vi "Test_WriteValue_InvalidRefnum_Error.vi"(8 "error in (no error)":errorcluster, 11 "TestCase in":refnum<class "TestTerminalCaptionBinding.lvclass">) -> (0 "error out":errorcluster, 3 "TestCase out":refnum<class "TestTerminalCaptionBinding.lvclass">)   [LabVIEW 2017, in "TestTerminalCaptionBinding.lvclass"]
uses:
  TestTerminalCaptionBinding.lvclass
  Source/Concrete/TerminalCaptionBinding/TerminalCaptionBinding.lvclass
  C:/Git/composed-transport/Source/ITransport/ITransport.lvclass
  Source/ITransport/ITransport.lvclass
panel:
  out "Return Error":errorcluster
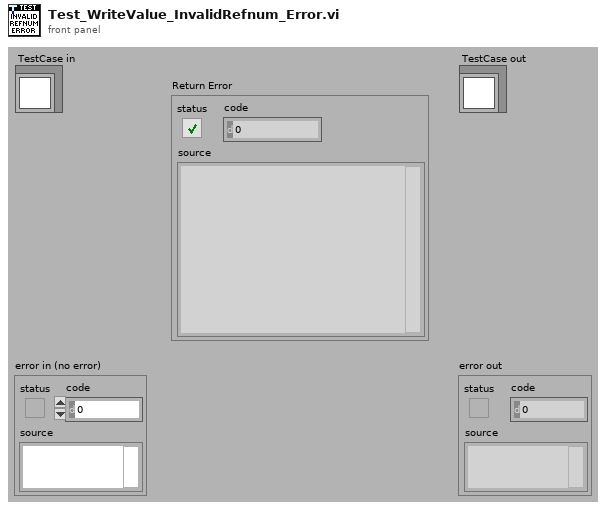
[diagram p1: front panel]
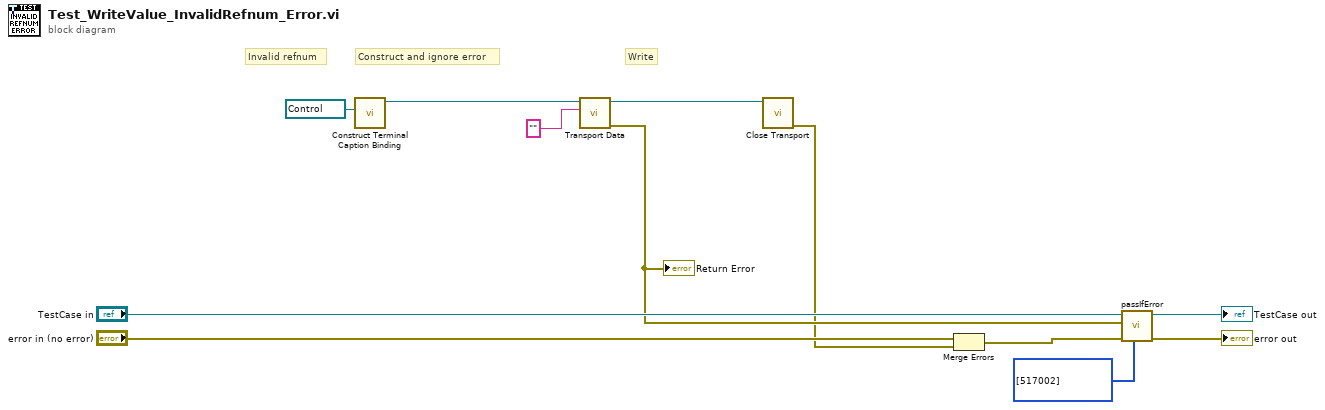
[diagram p0: block diagram]
diagram:
  # "Invalid refnum"
  # "Write"
  # "Construct and ignore error"
  n1 = call "Construct Terminal Caption Binding.vi"("Ctl Refnum"=refnum<vi> refnum) -> ("TerminalCaptionBinding"=w9:refnum<class "TerminalCaptionBinding.lvclass">)  [unwired: 9 in, 1 out]
  n2 = call "Transport Data.vi"("Value"="", "ITransport in"=w9) -> ("error out"=w7:errorcluster, "ITransport out"=w8:refnum<class "TerminalCaptionBinding.lvclass">)  [unwired: 8 in]
  "Return Error" <- w7
  n3 = call-dynamic "Close Transport.vi"("ITransport in"=w8) -> ("error out"=w1:errorcluster)  [unwired: 10 in]
  n4 = Merge Errors("error in (no error)", w1) -> (w4:errorcluster)
  n5 = call-dynamic "passIfError.vi"("passing error codes (default = any error code)"=i32[] [517002], "error in (no error)"=w4, "error"=w7, "TestCase in"="TestCase in") -> ("error out"=→"error out":errorcluster, "TestCase out"=→"TestCase out":refnum<class "TestTerminalCaptionBinding.lvclass">)  [unwired: 6 in]
